vi "tcpCmdArrayToZ_modify.vi"(7 "Delay (sec)":sgl[](array[numeric])=[0.0, 0.0, 0.0, 2.0, 0.0] format="%.2f", 8 "error in (no error)":errorcluster, 9 "Timeout (ms)":i32=40000000, 10 "Command array":string[](array[string])=["Hardware Control Layer", "Beamforming", "Common", "PulseVoltageA poke 1 2.00000E+1", "PulseVoltageA peek 1"], 11 "connection ID in":refnum<k5>) -> (0 "error out":errorcluster, 1 "Written-byte array":i32[](array[numeric])=[23, 12, 7, 32, 21], 2 "Receive array":string[](array[string])=["\r\n220 OK\r\nContainers within Hardware Control Layer\r\n\tHardwareModel\r\n\tHardwareControl\r\n\tHardwareAlgorithm\r\n\tSeq\r\n\tBeamforming\r\n\tDigitalReceiver\r\n\tEchoProcessor\r\n\tFlowProcessor\r\n\tHardwareScanConverter\r\n\tSip\r\n\tVideoInterface\r\n\tRtc\r\n\tCine\r\nScalar Parameters of Hardware Control Layer\r\nArray Parameters of Hardware Control Layer\r\ndebug\tDebug Functions\r\nquit\tExit DIOS\r\nback\tPrevious menu\r\nmain\tTop menu\r\nhelp\tAvailable commands\r\n\r\n", "\r\n220 OK\r\nContainers within Beamforming\r\n\tCommon\r\n\tBImage\r\n\tCbImage\r\n\tDImage\r\nScalar Parameters of Beamforming\r\nArray Parameters of Beamforming\r\ndebug\tDebug Functions\r\nquit\tExit DIOS\r\nback\tPrevious menu\r\nmain\tTop menu\r\nhelp\tAvailable commands\r\n\r\n", "\r\n220 OK\r\nContainers within Common\r\nScalar Parameters of Common\r\n\tBfPropagationVelCmPerSec\t154000\r\n\tDisUnit\t0.00385\r\n\tHwRcInterruptMask\t63\r\n\tHwRcTVP\t3\r\n\tHwRxAac0\t175\r\n\tHwRxAac1\t0\r\n\tHwRxbfBlankingWord\t0\r\n\tHwRxbfCmd1Word\t4232\r\n\tHwRxbfCmd2Word\t2\r\n\tHwRxbf0Cmd2Word\t3\r\n\tHwRxbfStartDelayWord\t10\r\n\tHwTiAttenuatorSelect\t0\r\n\tHwTiBitEn\t25088\r\n\tHwTiDacCtrl0\t255\r\n\tHwTiDacCtrl1\t2303\r\n\tHwTiDacCtrl2\t3327\r\n\tHwTiDacCtrl3\t511\r\n\tHwTiDacCtrl4\t2559\r\n\tHwTiDacCtrl5\t3583\r\n\tHwTiDacCtrl6\t767\r\n\tHwTiDacCtrl7\t2815\r\n\tHwTiDacCtrl8\t3839\r\n\tHwTiDacCtrl9\t2047\r\n\tHwTiDacCtrl10\t4095\r\n\tHwTiDigitalDriveCtrl\t0\r\n\tHwTiDigitalInterruptPolarity\t0\r\n\tHwTiDigitalReadCtrl\t0\r\n\tHwTiEchoBoosterCtrl\t0\r\n\tHwTiGlobalCtrl\t1\r\n\tHwTiHighVoltEn\t0\r\n\tHwTiInterruptClear\t65535\r\n\tHwTiInterruptMask\t32767\r\n\tHwTiMiscBitCtrl\t12\r\n\tHwTiProbeSelect\t2\r\n\tHwTiTXCLTransfer\t0\r\n\tHwTiVoltMultiplexer\t0\r\n\tHwTrGlobalCtrlAll\t1\r\n\tHwTrGlobalCtrl0All\t0\r\n\tHwTrDiagnosticCtrlAll\t0\r\n\tHwTrInterruptMaskAll\t1\r\n\tHwTrInterruptClearAll\t1\r\n\tHwTrRealTimeCtrlAll\t40\r\n\tHwTrTgcAacSignalCtrlAll\t0\r\n\tRxDelayRefx\t1\r\n\tRxDelayRefy\t-1\r\n\tTrPartNumber\t5928150\r\n\tBfPropagationVelFactor\t1\r\n\tDigitizingRateHz\t4e+007\r\n\tHwRxBfVectorLengthWord\t0\r\n\tIsRxVectorLengthEn\t1\r\n\tNumChannels\t192\r\n\tProbeBandwidthHz\t3.6e+006\r\n\tProbeId\t171\r\n\tProbeNumElem\t192\r\n\tProbeNumRows\t1\r\n\tProbePitchCm\t0.02\r\n\tProbeRadiusElectricalCm\t0\r\n\tProbeType\t0\r\n\tPropagationVelCmPerSec\t154000\r\n\tRxApod2dEn\t0\r\n\tRxbfAdcDelayClocks\t10\r\n\tRxbfGainShift\t0\r\n\tRxDelayYOffsetSysClk4\t0\r\n\tTxPulserMaxVolt\t50\r\nArray Parameters of Common\r\n\tHwRxbf0AdGainA\tsize=64\r\n\tHwRxbf1AdGainA\tsize=64\r\n\tHwRxbf2AdGainA\tsize=64\r\n\tHwRxbf3AdGainA\tsize=64\r\n\tHwRxbf4AdGainA\tsize=64\r\n\tHwRxbf5AdGainA\tsize=64\r\n\tHwRxbf6AdGainA\tsize=64\r\n\tHwRxbf7AdGainA\tsize=64\r\n\tHwRxbf8AdGainA\tsize=64\r\n\tHwRxbf9AdGainA\tsize=64\r\n\tHwRxbf10AdGainA\tsize=64\r\n\tHwRxbf11AdGainA\tsize=64\r\n\tHwRxAdOffsetCalA\tsize=192\r\n\tHwRxApodFilterRamA\tsize=512\r\n\tHwRxbf0DelayCalA\tsize=64\r\n\tHwRxbf1DelayCalA\tsize=64\r\n\tHwRxbf2DelayCalA\tsize=64\r\n\tHwRxbf3DelayCalA\tsize=64\r\n\tHwRxbf4DelayCalA\tsize=64\r\n\tHwRxbf5DelayCalA\tsize=64\r\n\tHwRxbf6DelayCalA\tsize=64\r\n\tHwRxbf7DelayCalA\tsize=64\r\n\tHwRxbf8DelayCalA\tsize=64\r\n\tHwRxbf9DelayCalA\tsize=64\r\n\tHwRxbf10DelayCalA\tsize=64\r\n\tHwRxbf11DelayCalA\tsize=64\r\n\tHwRxbf0DxA\tsize=64\r\n\tHwRxbf1DxA\tsize=64\r\n\tHwRxbf2DxA\tsize=64\r\n\tHwRxbf3DxA\tsize=64\r\n\tHwRxbf4DxA\tsize=64\r\n\tHwRxbf5DxA\tsize=64\r\n\tHwRxbf6DxA\tsize=64\r\n\tHwRxbf7DxA\tsize=64\r\n\tHwRxbf8DxA\tsize=64\r\n\tHwRxbf9DxA\tsize=64\r\n\tHwRxbf10DxA\tsize=64\r\n\tHwRxbf11DxA\tsize=64\r\n\tHwRxbf0DyA\tsize=64\r\n\tHwRxbf1DyA\tsize=64\r\n\tHwRxbf2DyA\tsize=64\r\n\tHwRxbf3DyA\tsize=64\r\n\tHwRxbf4DyA\tsize=64\r\n\tHwRxbf5DyA\tsize=64\r\n\tHwRxbf6DyA\tsize=64\r\n\tHwRxbf7DyA\tsize=64\r\n\tHwRxbf8DyA\tsize=64\r\n\tHwRxbf9DyA\tsize=64\r\n\tHwRxbf10DyA\tsize=64\r\n\tHwRxbf11DyA\tsize=64\r\n\tHwRxbf0DzA\tsize=128\r\n\tHwRxbf1DzA\tsize=128\r\n\tHwRxbf2DzA\tsize=128\r\n\tHwRxbf3DzA\tsize=128\r\n\tHwRxbf4DzA\tsize=128\r\n\tHwRxbf5DzA\tsize=128\r\n\tHwRxbf6DzA\tsize=128\r\n\tHwRxbf7DzA\tsize=128\r\n\tHwRxbf8DzA\tsize=128\r\n\tHwRxbf9DzA\tsize=128\r\n\tHwRxbf10DzA\tsize=128\r\n\tHwRxbf11DzA\tsize=128\r\n\tHwRxbf0PosInApodWinA\tsize=64\r\n\tHwRxbf1PosInApodWinA\tsize=64\r\n\tHwRxbf2PosInApodWinA\tsize=64\r\n\tHwRxbf3PosInApodWinA\tsize=64\r\n\tHwRxbf4PosInApodWinA\tsize=64\r\n\tHwRxbf5PosInApodWinA\tsize=64\r\n\tHwRxbf6PosInApodWinA\tsize=64\r\n\tHwRxbf7PosInApodWinA\tsize=64\r\n\tHwRxbf8PosInApodWinA\tsize=64\r\n\tHwRxbf9PosInApodWinA\tsize=64\r\n\tHwRxbf10PosInApodWinA\tsize=64\r\n\tHwRxbf11PosInApodWinA\tsize=64\r\n\tHwRxMuxSelectLutA\tsize=512\r\n\tHwRxRamOffsetA\tsize=12\r\n\tHwTxDacA\tsize=2\r\n\tHwTxpgDelayAperA\tsize=393216\r\n\tNumBitsPerCycleA\tsize=49\r\n\tNumCyclesPerPassA\tsize=49\r\n\tNumWordsPerPassA\tsize=49\r\n\tRxAdGainA\tsize=256\r\n\tRxDelayCalA\tsize=768\r\n\tRxDxA\tsize=256\r\n\tRxDyA\tsize=256\r\n\tRxDzA\tsize=256\r\n\tRxMuxSelectLutPtrA\tsize=512\r\n\tRxPosInApodWinA\tsize=768\r\n\tTxDelayCalA\tsize=192\r\n\tTxpgWaveformHoutA\tsize=15680\r\n\tTxpgWaveformLoutA\tsize=15680\r\n\tYIndexTableA\tsize=256\r\n\tZIndexTableA\tsize=256\r\n\tInsertedProbeIdA\tsize=6\r\n\tPulseVoltageA\tsize=2\r\n\tRxApodFactorA\tsize=4\r\n\tRxApodSelA\tsize=4\r\n\tSysTxFreqHzA\tsize=49\r\ndebug\tDebug Functions\r\nquit\tExit DIOS\r\nback\tPrevious menu\r\nmain\tTop menu\r\nhelp\tAvailable commands\r\n\r\n", "220 OK\r\n", "250 20\r\n"], 3 "connection ID out":refnum<k5>, 5 "Write/read times (ms)":u32[][](array[numeric])=[[0, 20, 22], [0, 10, 22], [1, 31, 23], [1, 11, 2023], [0, 10, 23]])   [LabVIEW 2016]
doc: "Sends an array of commands to the Z system, one at a time, via Telnet, and returns an array of Z system responses. The input array of delays should contain a delay time corresponding to each command. (Delays of 0 may be used for menu and read commands.) After each command is sent, the corresponding delay is waited out and then the response is read using tcpReadFromZ.vi"
uses:
  user/GrobaLimitVoltage.vi
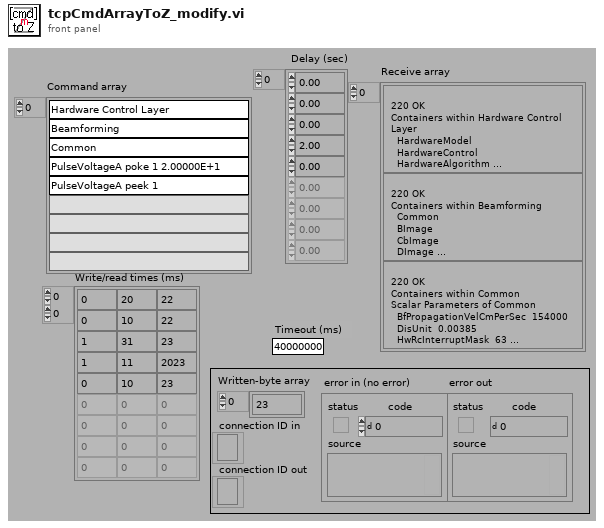
[diagram p1: front panel]
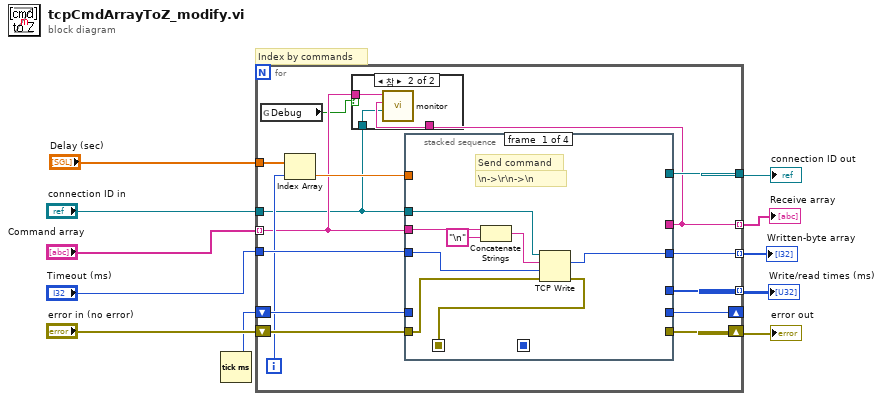
[diagram p0: block diagram]
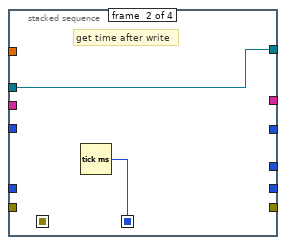
[diagram p3: hidden frame]
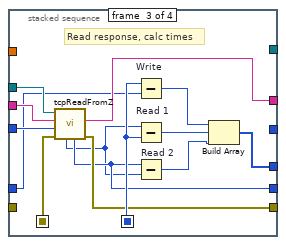
[diagram p4: hidden frame]
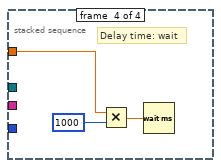
[diagram p5: hidden frame]
diagram:
  # "Index by commands"
  n1 = Tick Count (ms)() -> (millisecond timer value=w3:u32)
  n2 = for {
    shift-right: [w24] -> w8
    shift-left: "error in (no error)" -> [w26]
    tunnel: "connection ID in" -> [w13]
    tunnel: "Command array" -> [w15] mode=indexing
    tunnel: "Timeout (ms)" -> [w25]
    tunnel: [w23] -> w7 mode=indexing
    tunnel: [w14] -> w6 mode=indexing
    tunnel: [w22] -> w5 mode=indexing
    tunnel: [w21] -> w4
    shift-right: [w20] -> _
    shift-left: w3 -> [w19]
    tunnel: "Delay (sec)" -> [w18]
    i -> [w17]
    n3 = global read "GrobaLimitVoltage.vi" "Debug"() -> (w12:bool)
    n4 = Index Array(array=w18, index=w17) -> (element=w16:sgl)
    n5 = stacked-sequence {
      seq-local: [w35 _ _ _] -> [_ _ w53 _]
      seq-local: [_ w39 _ _] -> [_ _ w50 _]
      tunnel: [w34 _ _ _] -> w23
      tunnel: [_ _ w49 _] -> w22
      tunnel: [_ _ w43 _] -> w24
      tunnel: [_ _ w48 _] -> w14
      tunnel: w15 -> [w33 _ w47 _]
      tunnel: w25 -> [w32 _ w46 _]
      tunnel: w13 -> [w31 w38 w45 _]
      tunnel: w26 -> [w30 _ _ _]
      tunnel: [_ w38 _ _] -> w21
      tunnel: [_ _ w42 _] -> w20
      tunnel: w19 -> [_ _ w44 _]
      tunnel: w16 -> [_ _ _ w54]
      frame #0 {
        # "\\n->\\r\\n->\\n"
        # "Send command"
        n6 = Concatenate Strings(w33, "\n" ("Substring")) -> (w36:string)
        n7 = TCP Write(connection ID=w31, data in=w36, error in (no error)=w30, 9:w32) -> (bytes written=w34:i32, error out=w35:errorcluster)  [unwired: 1 out]
      }
      frame #1 {
        # "get time after write"
        n8 = Tick Count (ms)() -> (millisecond timer value=w39:u32)
      }
      frame #2 {
        # "Read response, calc times"
        n9 = call "tcpReadFromZ.vi"("error in (no error)"=w53, "Timeout (40000 ms)"=w46, "Command sent"=w47, "connection ID in"=w45) -> ("error out"=w43:errorcluster, "receive"=w48:string, "time 2 (ms)"=w42:u32, "time 1 (ms)"=w41:u32)  [unwired: 3 in, 1 out]
        n10 = Subtract "Write"(x=w50, y=w44) -> (x-y=w52:u32)
        n11 = Subtract "Read 1"(x=w41, y=w50) -> (x-y=w51:u32)
        n12 = Subtract "Read 2"(x=w42, y=w41) -> (x-y=w40:u32)
        n13 = Build Array(w52, w51, w40) -> (w49:u32[])
      }
      frame #3 {
        # "Delay time: wait"
        n14 = Multiply(x=w54, y=u32 1000) -> (x*y=w56:sgl)
        n15 = Wait (ms)(milliseconds to wait=w56) -> ()  [unwired: 1 out]
      }
    }
    n16 = case shown="참" w12 {
      tunnel: w15 -> [_ w29]
      tunnel: w14 -> [_ w28]
      tunnel: w13 -> [_ w27]
      frame False {
      }
      frame True {
        n17 = call "monitor.vi"("connection ID in"=w27, "Received text 4"=w28, "Received text 2"=w29) -> ()  [unwired: 3 in]
      }
    }
  }
  "connection ID out" <- w4
  "Receive array" <- w6
  "Written-byte array" <- w7
  "Write/read times (ms)" <- w5
  "error out" <- w8
